vi "Read PRACH Modulation EVM Power Vs Preamble Results.vi"(0 "VISA resource name":refnum<visa-resource-name>, 5 "Instance (1)":T2=1, 7 "Preamble (1)":T1=1, 11 "error in (no error)":errorcluster) -> (4 "VISA resource name out":refnum<visa-resource-name>, 6 "Reliability":i32, 8 "Out Of Tolerance":i32, 10 "Results":dbl[](array[numeric]) format="%^.3e", 15 "error out":errorcluster)   [LabVIEW 2020, in "Rohde&Schwarz CMWXP NR FR1 Measurement.lvlib"]
doc: "Starts a new single shot measurement and returns the single value results of the 'EVM vs Preamble' and 'Power vs Preamble' squares, for a selected preamble.\n\nAttribute:\nRSCMWXPNRFR1M_ATTR_READ_PRACH_MODULATION_EVM_POWER_VS_PREAMBLE_RESULTS\n\nRemote-control command:\nREAD:NRSub:MEAS<i>:PRACh:MODulation:PREamble<Number>?"
uses:
  <instrlib>/Rohde&Schwarz CMWXP NR FR1 Measurement/Rohde&Schwarz CMWXP NR FR1 Measurement.lvlib
  <instrlib>/Rohde&Schwarz CMWXP NR FR1 Measurement/Private/_Instance.ctl
  <instrlib>/Rohde&Schwarz CMWXP NR FR1 Measurement/Private/_Preamble.ctl
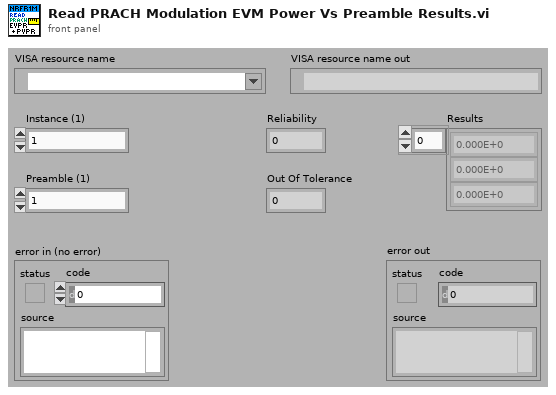
[diagram p1: front panel]
types:
  T1 = typedef "Rohde&Schwarz CMWXP NR FR1 Measurement.lvlib/_Preamble.ctl" = i32
  T2 = typedef "Rohde&Schwarz CMWXP NR FR1 Measurement.lvlib/_Instance.ctl" = i32
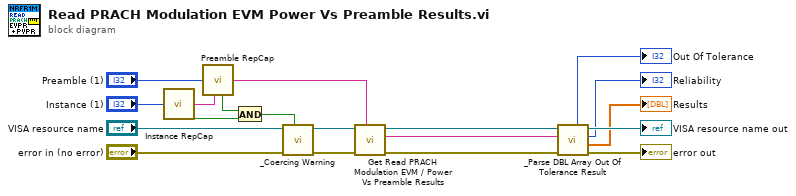
[diagram p0: block diagram]
diagram:
  n1 = call <instrlib>:"Instance RepCap.vi"("Instance In"="Instance (1)") -> ("In Range?"=w15:bool, "RepCap Identifier Out"=w16:string)  [unwired: 1 in]
  n2 = call <instrlib>:"Preamble RepCap.vi"("Preamble In"="Preamble (1)", "RepCap String In (\"\")"=w16) -> ("In Range?"=w14:bool, "RepCap Identifier Out"=w1:string)
  n3 = And(x=w14, y=w15) -> (x .and. y?=w11:bool)
  n4 = call <instrlib>:"_Coercing Warning.vi"("In Range?"=w11, "error in (no error)"="error in (no error)", "VISA resource name"="VISA resource name") -> ("error out"=w17:errorcluster, "VISA resource name out"=w10:refnum<visa-resource-name>)  [unwired: 7 in]
  n5 = call "Get Read PRACH Modulation EVM / Power Vs Preamble Results"("Repeated Capabilities"=w1, "error in (no error)"=w17, "instrument handle"=w10) -> ("error out"=w9:errorcluster, "Read PRACH Modulation EVM / Power Vs Preamble Results"=w8:string, "instrument handle out"=w7:refnum<visa-resource-name>)  [unwired: 6 in]
  n6 = call <instrlib>:"_Parse DBL Array Out Of Tolerance Result.vi"("error in (no error)"=w9, "Input String"=w8, "VISA resource name"=w7) -> ("error out"=→"error out":errorcluster, "Results"=→"Results":dbl[], "Reliability"=→"Reliability":i32, "VISA resource name out"=→"VISA resource name out":refnum<visa-resource-name>, "Out Of Tolerance"=→"Out Of Tolerance":i32)  [unwired: 4 in]
